vi "Unescape String.vi"(5 "Unescape? [T]":bool=TRUE, 8 "error in (no error)":errorcluster, 10 "String":string, 11 "Registry Object":refnum<class "Carya Config.lvclass">) -> (0 "error out":errorcluster, 2 "Unescaped string":string, 3 "Registry Object":refnum<class "Carya Config.lvclass">)   [LabVIEW 2013, in "Carya Config.lvclass"]
doc: "Copyright 2018, Carya Automatisering, Wiebe Walstra."
uses:
  Carya Config.lvclass
  <vilib>/regexp/Match Regular Expression.xnode
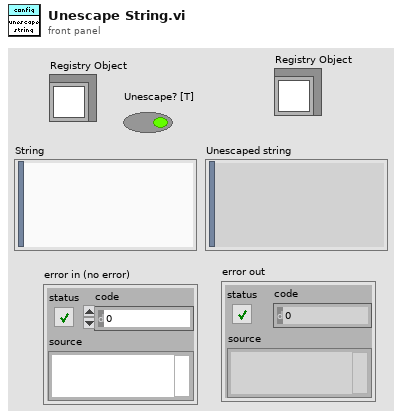
[diagram p1: front panel]
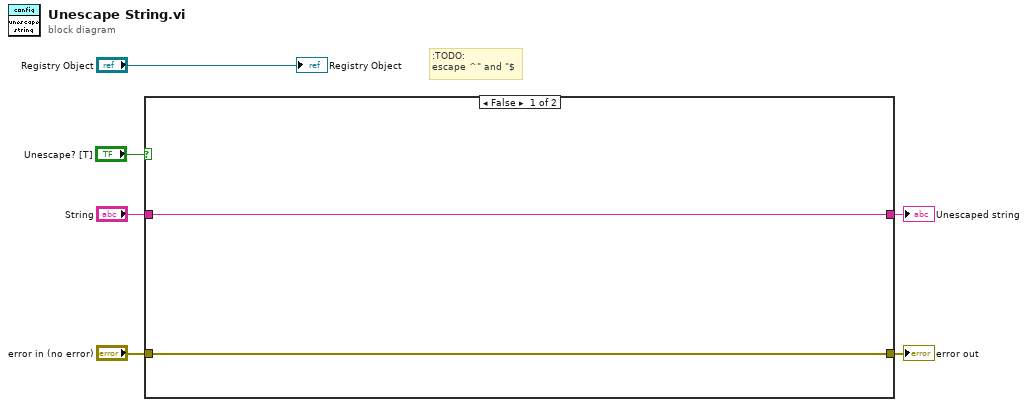
[diagram p0: block diagram]
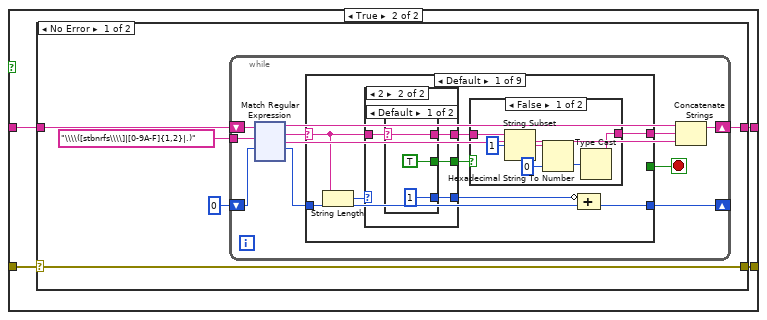
[diagram p2: hidden frame]
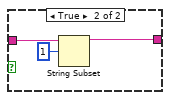
[diagram p3: hidden frame]
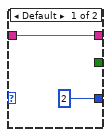
[diagram p4: hidden frame]
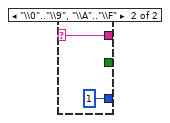
[diagram p5: hidden frame]
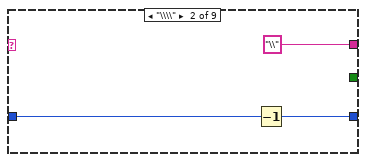
[diagram p6: hidden frame]
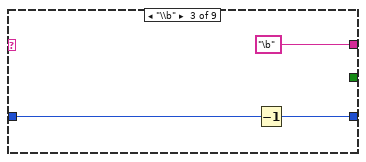
[diagram p7: hidden frame]
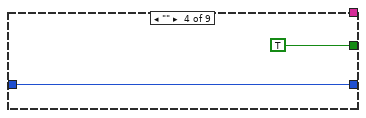
[diagram p8: hidden frame]
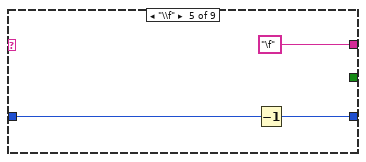
[diagram p9: hidden frame]
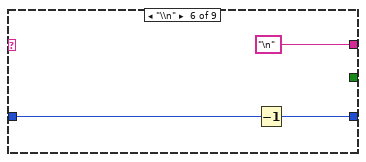
[diagram p10: hidden frame]
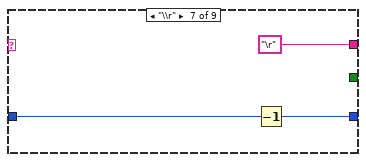
[diagram p11: hidden frame]
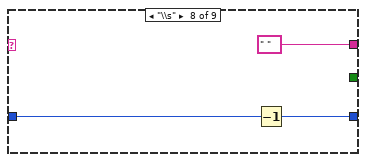
[diagram p12: hidden frame]
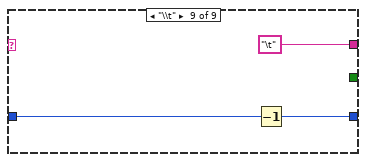
[diagram p13: hidden frame]
diagram:
  # ":TODO:\nescape ^\" and \"$"
  n1 = case shown="False" "Unescape? [T]" {
    tunnel: "String" -> [w8 w12]
    tunnel: [w8 w11] -> w4
    tunnel: "error in (no error)" -> [w7 w10]
    tunnel: [w7 w9] -> w2
    frame False {
    }
    frame True {
      n2 = case shown="No Error" w10 {
        selector: w10 -> [w13 w194]
        tunnel: w12 -> [w15 _]
        tunnel: [w14 _] -> w11
        tunnel: [w13 w194] -> w9
        frame No Error {
          n3 = while {
            tunnel: "\\\\([stbnrfs\\\\]|[0-9A-F]{1,2}|.)" ("regular expression") -> [w27]
            shift-right: [w24] -> w14
            shift-left: w15 -> [w28]
            shift-right: [w19] -> _
            shift-left: 0 ("offset past match") -> [w21]
            stop <- w18 stop-if-true
            n4 = xnode "Match Regular Expression"("input string"=w28, "regular expression"=w27, "offset (0)"=w21) -> ("before match"=w23:string, "whole match"=w26:string, "after match"=w22:string, "offset past match"=w20:i32)  [unwired: 3 in, 1 out]
            n5 = case shown="Default" w26 {
              selector: w26 -> [w31 _ _ _ _ _ _ _ _]
              tunnel: [w36 "\\" "\b" _ "\f" "\n" "\r" " " "\t"] -> w25
              tunnel: w20 -> [w35 w58 w61 w64 w66 w69 w72 w75 w78]
              tunnel: [w34 w57 w60 w64 w65 w68 w71 w74 w77] -> w19
              tunnel: [_ _ _ TRUE _ _ _ _ _] -> w18
              frame Default {
                n6 = String Length(string=w31) -> (length=w33:i32)
                n7 = case shown="2" w33 {
                  tunnel: [w47 w50] -> w32
                  tunnel: w31 -> [w47 w51]
                  tunnel: [_ w49] -> w30
                  tunnel: [2 w48] -> w29
                  frame Default {
                  }
                  frame 2 {
                    n8 = case shown="Default" w51 {
                      selector: w51 -> [w54 w56]
                      tunnel: [w54 w56] -> w50
                      tunnel: [TRUE _] -> w49
                      tunnel: [1 1] -> w48
                      frame Default {
                      }
                      frame "\\0".."\\9", "\\A".."\\F" {
                      }
                    }
                  }
                }
                n9 = case shown="False" w30 {
                  tunnel: [w42 w43] -> w36
                  tunnel: w32 -> [w37 w45]
                  frame False {
                    n10 = String Subset(string=w37, offset (0)=1) -> (substring=w38:string)  [unwired: 1 in]
                    n11 = Hexadecimal String To Number(string=w38, default (0uL)=u8 0 ("default (0 U32)")) -> (number=w39:u8)  [unwired: 1 in, 1 out]
                    n12 = Type Cast(x=w39) -> (*(type *) &x=w42:string)  [unwired: 1 in]
                  }
                  frame True {
                    n13 = String Subset(string=w45, offset (0)=1) -> (substring=w43:string)  [unwired: 1 in]
                  }
                }
                n14 = Compound Arithmetic op=ADD(invert w29, w35) -> (w34:i32)
              }
              frame "\\\\" {
                n15 = Decrement(x=w58) -> (x-1=w57:i32)
              }
              frame "\\b" {
                n16 = Decrement(x=w61) -> (x-1=w60:i32)
              }
              frame "" {
              }
              frame "\\f" {
                n17 = Decrement(x=w66) -> (x-1=w65:i32)
              }
              frame "\\n" {
                n18 = Decrement(x=w69) -> (x-1=w68:i32)
              }
              frame "\\r" {
                n19 = Decrement(x=w72) -> (x-1=w71:i32)
              }
              frame "\\s" {
                n20 = Decrement(x=w75) -> (x-1=w74:i32)
              }
              frame "\\t" {
                n21 = Decrement(x=w78) -> (x-1=w77:i32)
              }
            }
            n22 = Concatenate Strings(w23, w25, w22) -> (w24:string)
          }
        }
        frame Error {
        }
      }
    }
  }
  "error out" <- w2
  "Unescaped string" <- w4
  "Registry Object" <- "Registry Object"
